vi "Sort_TC_Data.vi"(10 "TC_data":dbl[](array[numeric]), 11 "AlarmSettings":T1={"TC13"={"Enbl"=FALSE, "ErrsAndWarns"={0.0, 5.663716814159292, 7.168141592920354, 8.584070796460177}}, "AI1"={"Enbl"=FALSE, "ErrsAndWarns"={0.0, 5.663716814159292, 7.168141592920354, 8.584070796460177}}, "AI2"={"Enbl"=FALSE, "ErrsAndWarns"={0.0, 5.663716814159292, 7.168141592920354, 8.584070796460177}}, "AI3"={"Enbl"=FALSE, "ErrsAndWarns"={0.0, 5.663716814159292, 7.168141592920354, 8.584070796460177}}, "AI4"={"Enbl"=FALSE, "ErrsAndWarns"={0.0, 5.663716814159292, 7.168141592920354, 8.584070796460177}}, "AI5"={"Enbl"=FALSE, "ErrsAndWarns"={0.0, 5.663716814159292, 7.168141592920354, 8.584070796460177}}, "AI6"={"Enbl"=FALSE, "ErrsAndWarns"={0.0, 5.663716814159292, 7.168141592920354, 8.584070796460177}}, "AI18"={"Enbl"=FALSE, "ErrsAndWarns"={0.0, 5.663716814159292, 7.168141592920354, 8.584070796460177}}, "AI19"={"Enbl"=FALSE, "ErrsAndWarns"={0.0, 5.663716814159292, 7.168141592920354, 8.584070796460177}}, "TE1"={"Enbl"=FALSE, "ErrsAndWarns"={0.0, 5.663716814159292, 7.168141592920354, 8.584070796460177}}, "TE2"={"Enbl"=FALSE, "ErrsAndWarns"={0.0, 5.663716814159292, 7.168141592920354, 8.584070796460177}}, "TE3"={"Enbl"=FALSE, "ErrsAndWarns"={0.0, 5.663716814159292, 7.168141592920354, 8.584070796460177}}, "ADAM1"={"Enbl"=FALSE, "ErrsAndWarns"={0.0, 5.663716814159292, 7.168141592920354, 8.584070796460177}}, "ADAM2"={"Enbl"=FALSE, "ErrsAndWarns"={0.0, 5.663716814159292, 7.168141592920354, 8.584070796460177}}, "ADAM3"={"Enbl"=FALSE, "ErrsAndWarns"={0.0, 5.663716814159292, 7.168141592920354, 8.584070796460177}}, "ADAM4"={"Enbl"=FALSE, "ErrsAndWarns"={0.0, 5.663716814159292, 7.168141592920354, 8.584070796460177}}, "72CoBeacFreq"={"Enbl"=FALSE, "ErrsAndWarns"={0.0, 5.663716814159292, 7.168141592920354, 8.584070796460177}}, "72CoCalFreq"={"Enbl"=FALSE, "ErrsAndWarns"={0.0, 5.663716814159292, 7.168141592920354, 8.584070796460177}}, "84CoBeacFreq"={"Enbl"=FALSE, "ErrsAndWarns"={0.0, 5.663716814159292, 7.168141592920354, 8.584070796460177}}, "84CoCalFreq"={"Enbl"=FALSE, "ErrsAndWarns"={0.0, 5.663716814159292, 7.168141592920354, 8.584070796460177}}, "72Co_CalTonePwr"={"Enbl"=FALSE, "ErrsAndWarns"={0.0, 5.663716814159292, 7.168141592920354, 8.584070796460177}}, "72X_CalTonePwr"={"Enbl"=FALSE, "ErrsAndWarns"={0.0, 5.663716814159292, 7.168141592920354, 8.584070796460177}}, "84Co_CalTonePwr"={"Enbl"=FALSE, "ErrsAndWarns"={0.0, 5.663716814159292, 7.168141592920354, 8.584070796460177}}, "84X_CalTonePwr"={"Enbl"=FALSE, "ErrsAndWarns"={0.0, 5.663716814159292, 7.168141592920354, 8.584070796460177}}} {"84X_CalTonePwr"."ErrsAndWarns" scale=-120.0..-45.0; "72X_CalTonePwr"."ErrsAndWarns" scale=-120.0..-45.0; "84Co_CalTonePwr"."ErrsAndWarns" scale=-120.0..-45.0; "72Co_CalTonePwr"."ErrsAndWarns" scale=-120.0..-45.0; "84CoCalFreq"."ErrsAndWarns" scale=24.9..25.1; "84CoBeacFreq"."ErrsAndWarns" scale=25.5..27.0; "72CoCalFreq"."ErrsAndWarns" scale=24.9..25.1; "72CoBeacFreq"."ErrsAndWarns" scale=25.5..27.0; "ADAM4"."ErrsAndWarns" scale=30.0..52.0; "ADAM3"."ErrsAndWarns" scale=30.0..52.0; "ADAM2"."ErrsAndWarns" scale=30.0..52.0; "ADAM1"."ErrsAndWarns" scale=30.0..52.0; "TE3"."ErrsAndWarns" scale=30.0..52.0; "TE2"."ErrsAndWarns" scale=30.0..52.0; "TE1"."ErrsAndWarns" scale=20.0..52.0; "AI19"."ErrsAndWarns" scale=0.0..60.0; "AI18"."ErrsAndWarns" scale=-10.0..10.0; "AI6"."ErrsAndWarns" scale=0.0..35.0; "AI5"."ErrsAndWarns" scale=0.0..20.0; "AI4"."ErrsAndWarns" scale=0.0..15.0; "AI3"."ErrsAndWarns" scale=0.0..10.0; "AI2"."ErrsAndWarns" scale=0.0..10.0; "TC13"."ErrsAndWarns" scale=-10.0..40.0}) -> (3 "TC_Variant":variant)   [LabVIEW 2018]
uses:
  Controls/Clusts/AlarmSettingsClust.ctl
  Controls/Clusts/AlarmThresh_OneChan.ctl
  HDF5/TC_Data_Structure.ctl
  Controls/Clusts/All_TC_Error_Status.ctl
  Controls/Clusts/ErrorStatus.ctl
  Controls/Clusts/All_TC_Error_and_Data.ctl
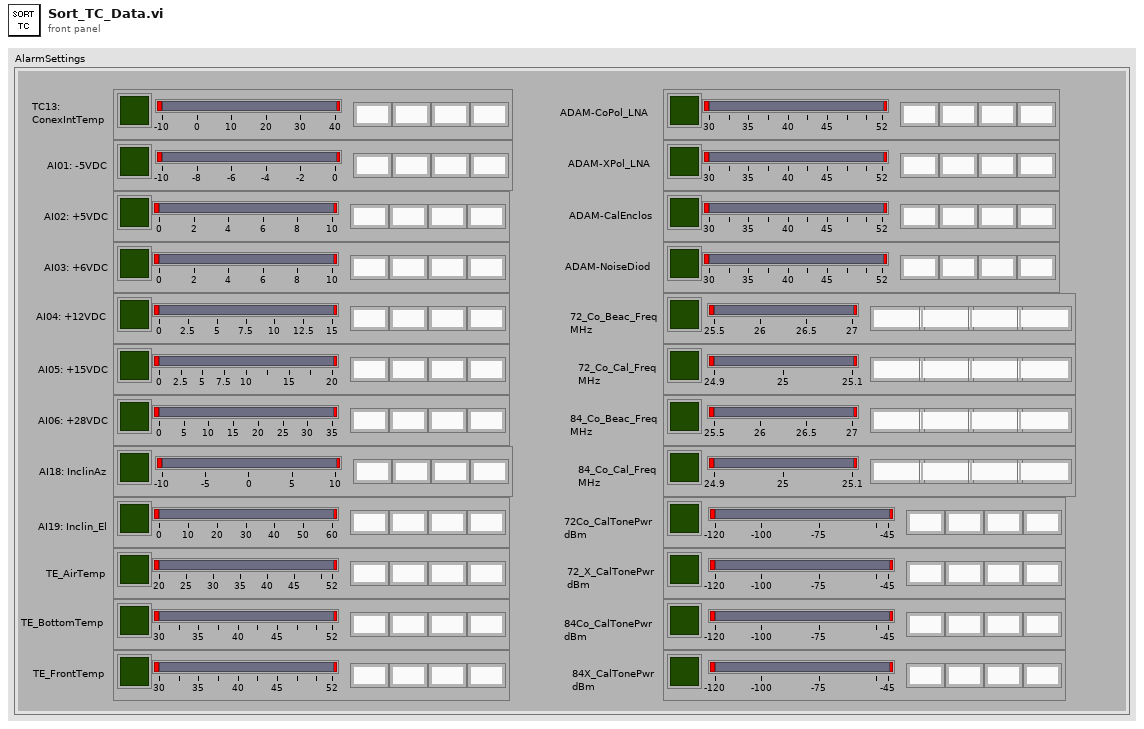
[diagram p1: front panel]
types:
  T1 = typedef "AlarmSettingsClust.ctl" = cluster{"TC13":T2, "AI1":T2, "AI2":T2, "AI3":T2, "AI4":T2, "AI5":T2, "AI6":T2, "AI18":T2, "AI19":T2, "TE1":T2, "TE2":T2, "TE3":T2, "ADAM1":T2, "ADAM2":T2, "ADAM3":T2, "ADAM4":T2, "72CoBeacFreq":T2, "72CoCalFreq":T2, "84CoBeacFreq":T2, "84CoCalFreq":T2, "72Co_CalTonePwr":T2, "72X_CalTonePwr":T2, "84Co_CalTonePwr":T2, "84X_CalTonePwr":T2}
  T2 = typedef "AlarmThresh_OneChan.ctl" = cluster{"Enbl":bool, "ErrsAndWarns":cluster{dbl, dbl, dbl, dbl}}
  T3 = typedef "All_TC_Error_and_Data.ctl" = cluster{"TCData":T4, "All_TC_ErrorStatus":T5}
  T4 = typedef "TC_Data_Structure.ctl" = cluster{"TimeStamp":dbl, "TimeString":string, "TC0_LP1_Hi":dbl, "TC1_LP1_MidHi":dbl, "TC2_LP1_Mid":dbl, "TC3_LP1_LoMid":dbl, "TC4_LP1_Lo":dbl, "TC5_LP2_Hi":dbl, "TC6_LP2_MidHi":dbl, "TC7_LP2_Mid":dbl, "TC8_LP2_LoMid":dbl, "TC9_LP2_Lo":dbl, "TC10_HVAC_Cond_In":dbl, "TC11_HVAC_Cond_Out":dbl, "TC12_Gen_Exhaust":dbl, "TC13_Amb_Inter":dbl, "TC14_Unused":dbl, "TC15_Unused":dbl, "TC16_Unused":dbl, "TC17_Unused":dbl, "TC18_Unused":dbl, "TC19_Unused":dbl, "TC20_Unused":dbl, "TC21_Unused":dbl, "TC22_Unused":dbl, "TC23_Unused":dbl, "TC24_Unused":dbl, "TC25_Unused":dbl, "TC26_Unused":dbl, "TC27_Unused":dbl, "TC28_Unused":dbl, "TC29_Unused":dbl, "TC30_Unused":dbl, "TC31_Unused":dbl}
  T5 = typedef "All_TC_Error_Status.ctl" = cluster{"TC 0":T6, "TC 1":T6, "TC 2":T6, "TC 3":T6, "TC 4":T6, "TC 5":T6, "TC 6":T6, "TC 7":T6, "TC 8":T6, "TC 9":T6, "TC 10":T6, "TC 11":T6, "TC 12":T6, "TC 13":T6, "TC 14":T6, "TC 15":T6, "TC 16":T6, "TC 17":T6, "TC 18":T6, "TC 19":T6, "TC 20":T6}
  T6 = typedef "ErrorStatus.ctl" = cluster{"RX?":bool, "Warn":bool, "Error":bool, "Enabl":bool, "Source":string}
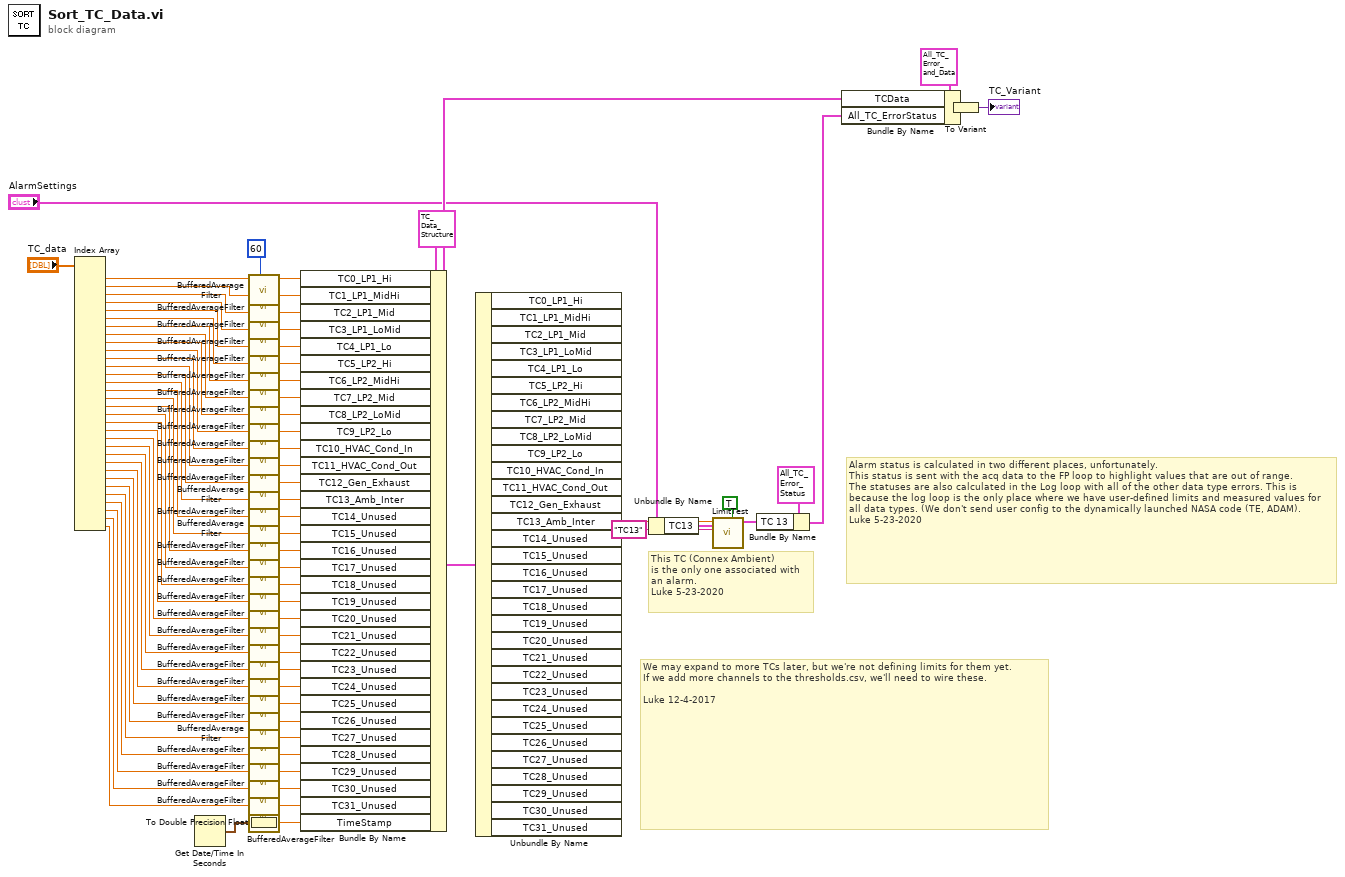
[diagram p0: block diagram]
diagram:
  w51 = 60 ("Buffer Size")
  # "This TC (Connex Ambient)\nis the only one associated with\nan alarm.\nLuke 5-23-2020"
  # "Alarm status is calculated in two different places, unfortunately.\nThis status is sent with the acq data to the FP loop to highlight values that are out of range.\nThe statuses are also calculated in the Log loop with all of the other data type errors. This is because the log loop is the only place where we have user-defined limits and measured values for all data types. (We don't send user config to the dynamically launched NASA code (TE, ADAM). \nLuke 5-23-2020"
  # "We may expand to more TCs later, but we're not defining limits for them yet.\nIf we add more channels to the thresholds.csv, we'll need to wire these.\n\nLuke 12-4-2017"
  n1 = Index Array(array="TC_data") -> (element #1=w70:dbl, element #2=w69:dbl, element #3=w68:dbl, element #4=w67:dbl, element #5=w66:dbl, element #6=w65:dbl, element #7=w64:dbl, element #8=w63:dbl, element #9=w62:dbl, element #10=w61:dbl, element #11=w60:dbl, element #12=w59:dbl, element #13=w58:dbl, element #14=w57:dbl, element #15=w56:dbl, element #16=w55:dbl, element #17=w54:dbl, element #18=w53:dbl, element #19=w52:dbl, element #20=w50:dbl, element #21=w49:dbl, element #22=w48:dbl, element #23=w47:dbl, element #24=w46:dbl, element #25=w45:dbl, element #26=w44:dbl, element #27=w43:dbl, element #28=w42:dbl, element #29=w41:dbl, element #30=w40:dbl, element #31=w39:dbl, element #32=w38:dbl)  [unwired: 32 in]
  n2 = Get Date/Time In Seconds() -> (seconds since 1Jan1904=w1:timestamp)
  n3 = call "BufferedAverageFilter.vi"("Buffer Size"=w51, "Signal"=w70) -> ("FilteredSignal"=w37:dbl)  [unwired: 9 in]
  n4 = call "BufferedAverageFilter.vi"("Buffer Size"=w51, "Signal"=w69) -> ("FilteredSignal"=w36:dbl)  [unwired: 9 in]
  n5 = call "BufferedAverageFilter.vi"("Buffer Size"=w51, "Signal"=w68) -> ("FilteredSignal"=w35:dbl)  [unwired: 9 in]
  n6 = call "BufferedAverageFilter.vi"("Buffer Size"=w51, "Signal"=w67) -> ("FilteredSignal"=w34:dbl)  [unwired: 9 in]
  n7 = call "BufferedAverageFilter.vi"("Buffer Size"=w51, "Signal"=w66) -> ("FilteredSignal"=w33:dbl)  [unwired: 9 in]
  n8 = call "BufferedAverageFilter.vi"("Buffer Size"=w51, "Signal"=w65) -> ("FilteredSignal"=w32:dbl)  [unwired: 9 in]
  n9 = call "BufferedAverageFilter.vi"("Buffer Size"=w51, "Signal"=w64) -> ("FilteredSignal"=w31:dbl)  [unwired: 9 in]
  n10 = call "BufferedAverageFilter.vi"("Buffer Size"=w51, "Signal"=w63) -> ("FilteredSignal"=w30:dbl)  [unwired: 9 in]
  n11 = call "BufferedAverageFilter.vi"("Buffer Size"=w51, "Signal"=w62) -> ("FilteredSignal"=w29:dbl)  [unwired: 9 in]
  n12 = call "BufferedAverageFilter.vi"("Buffer Size"=w51, "Signal"=w61) -> ("FilteredSignal"=w28:dbl)  [unwired: 9 in]
  n13 = call "BufferedAverageFilter.vi"("Buffer Size"=w51, "Signal"=w60) -> ("FilteredSignal"=w27:dbl)  [unwired: 9 in]
  n14 = call "BufferedAverageFilter.vi"("Buffer Size"=w51, "Signal"=w59) -> ("FilteredSignal"=w26:dbl)  [unwired: 9 in]
  n15 = call "BufferedAverageFilter.vi"("Buffer Size"=w51, "Signal"=w58) -> ("FilteredSignal"=w25:dbl)  [unwired: 9 in]
  n16 = call "BufferedAverageFilter.vi"("Buffer Size"=w51, "Signal"=w57) -> ("FilteredSignal"=w24:dbl)  [unwired: 9 in]
  n17 = call "BufferedAverageFilter.vi"("Buffer Size"=w51, "Signal"=w56) -> ("FilteredSignal"=w23:dbl)  [unwired: 9 in]
  n18 = call "BufferedAverageFilter.vi"("Buffer Size"=w51, "Signal"=w55) -> ("FilteredSignal"=w22:dbl)  [unwired: 9 in]
  n19 = call "BufferedAverageFilter.vi"("Buffer Size"=w51, "Signal"=w54) -> ("FilteredSignal"=w21:dbl)  [unwired: 9 in]
  n20 = call "BufferedAverageFilter.vi"("Buffer Size"=w51, "Signal"=w53) -> ("FilteredSignal"=w20:dbl)  [unwired: 9 in]
  n21 = call "BufferedAverageFilter.vi"("Buffer Size"=w51, "Signal"=w52) -> ("FilteredSignal"=w19:dbl)  [unwired: 9 in]
  n22 = call "BufferedAverageFilter.vi"("Buffer Size"=w51, "Signal"=w50) -> ("FilteredSignal"=w18:dbl)  [unwired: 9 in]
  n23 = call "BufferedAverageFilter.vi"("Buffer Size"=w51, "Signal"=w49) -> ("FilteredSignal"=w17:dbl)  [unwired: 9 in]
  n24 = call "BufferedAverageFilter.vi"("Buffer Size"=w51, "Signal"=w48) -> ("FilteredSignal"=w16:dbl)  [unwired: 9 in]
  n25 = call "BufferedAverageFilter.vi"("Buffer Size"=w51, "Signal"=w47) -> ("FilteredSignal"=w15:dbl)  [unwired: 9 in]
  n26 = call "BufferedAverageFilter.vi"("Buffer Size"=w51, "Signal"=w46) -> ("FilteredSignal"=w14:dbl)  [unwired: 9 in]
  n27 = call "BufferedAverageFilter.vi"("Buffer Size"=w51, "Signal"=w45) -> ("FilteredSignal"=w13:dbl)  [unwired: 9 in]
  n28 = call "BufferedAverageFilter.vi"("Buffer Size"=w51, "Signal"=w44) -> ("FilteredSignal"=w12:dbl)  [unwired: 9 in]
  n29 = call "BufferedAverageFilter.vi"("Buffer Size"=w51, "Signal"=w43) -> ("FilteredSignal"=w11:dbl)  [unwired: 9 in]
  n30 = call "BufferedAverageFilter.vi"("Buffer Size"=w51, "Signal"=w42) -> ("FilteredSignal"=w10:dbl)  [unwired: 9 in]
  n31 = call "BufferedAverageFilter.vi"("Buffer Size"=w51, "Signal"=w41) -> ("FilteredSignal"=w9:dbl)  [unwired: 9 in]
  n32 = call "BufferedAverageFilter.vi"("Buffer Size"=w51, "Signal"=w40) -> ("FilteredSignal"=w8:dbl)  [unwired: 9 in]
  n33 = call "BufferedAverageFilter.vi"("Buffer Size"=w51, "Signal"=w39) -> ("FilteredSignal"=w7:dbl)  [unwired: 9 in]
  n34 = call "BufferedAverageFilter.vi"("Buffer Size"=w51, "Signal"=w38) -> ("FilteredSignal"=w6:dbl)  [unwired: 9 in]
  n35 = To Double Precision Float(number=w1) -> (double precision float=w2:dbl)
  n36 = Bundle By Name(cluster=T4 {"TimeStamp"=0.0, "TimeString"="", "TC0_LP1_Hi"=0.0, "TC1_LP1_MidHi"=0.0, "TC2_LP1_Mid"=0.0, "TC3_LP1_LoMid"=0.0, "TC4_LP1_Lo"=0.0, "TC5_LP2_Hi"=0.0, "TC6_LP2_MidHi"=0.0, "TC7_LP2_Mid"=0.0, "TC8_LP2_LoMid"=0.0, "TC9_LP2_Lo"=0.0, "TC10_HVAC_Cond_In"=0.0, "TC11_HVAC_Cond_Out"=0.0, "TC12_Gen_Exhaust"=0.0, "TC13_Amb_Inter"=0.0, "TC14_Unused"=0.0, "TC15_Unused"=0.0, "TC16_Unused"=0.0, "TC17_Unused"=0.0, "TC18_Unused"=0.0, "TC19_Unused"=0.0, "TC20_Unused"=0.0, "TC21_Unused"=0.0, "TC22_Unused"=0.0, "TC23_Unused"=0.0, "TC24_Unused"=0.0, "TC25_Unused"=0.0, "TC26_Unused"=0.0, "TC27_Unused"=0.0, "TC28_Unused"=0.0, "TC29_Unused"=0.0, "TC30_Unused"=0.0, "TC31_Unused"=0.0} ("TCData"), "TC0_LP1_Hi"=w37, "TC1_LP1_MidHi"=w36, "TC2_LP1_Mid"=w35, "TC3_LP1_LoMid"=w34, "TC4_LP1_Lo"=w33, "TC5_LP2_Hi"=w32, "TC6_LP2_MidHi"=w31, "TC7_LP2_Mid"=w30, "TC8_LP2_LoMid"=w29, "TC9_LP2_Lo"=w28, "TC10_HVAC_Cond_In"=w27, "TC11_HVAC_Cond_Out"=w26, "TC12_Gen_Exhaust"=w25, "TC13_Amb_Inter"=w24, "TC14_Unused"=w23, "TC15_Unused"=w22, "TC16_Unused"=w21, "TC17_Unused"=w20, "TC18_Unused"=w19, "TC19_Unused"=w18, "TC20_Unused"=w17, "TC21_Unused"=w16, "TC22_Unused"=w15, "TC23_Unused"=w14, "TC24_Unused"=w13, "TC25_Unused"=w12, "TC26_Unused"=w11, "TC27_Unused"=w10, "TC28_Unused"=w9, "TC29_Unused"=w8, "TC30_Unused"=w7, "TC31_Unused"=w6, "TimeStamp"=w2) -> (w73:T4)
  n37 = Unbundle By Name(w73) -> ("TC13_Amb_Inter"=w77:dbl)  [unwired: 31 out]
  n38 = Unbundle By Name("AlarmSettings") -> ("TC13"=w78:T2)
  n39 = call "LimitTest.vi"("RX?"=TRUE, "AlarmCfg"=w78, "Source"="TC13", "Data"=w77) -> ("ErrorStatus"=w75:T6)  [unwired: 7 in]
  n40 = Bundle By Name(cluster=T5 {"TC 0"={"RX?"=FALSE, "Warn"=FALSE, "Error"=FALSE, "Enabl"=FALSE, "Source"=""}, "TC 1"={"RX?"=FALSE, "Warn"=FALSE, "Error"=FALSE, "Enabl"=FALSE, "Source"=""}, "TC 2"={"RX?"=FALSE, "Warn"=FALSE, "Error"=FALSE, "Enabl"=FALSE, "Source"=""}, "TC 3"={"RX?"=FALSE, "Warn"=FALSE, "Error"=FALSE, "Enabl"=FALSE, "Source"=""}, "TC 4"={"RX?"=FALSE, "Warn"=FALSE, "Error"=FALSE, "Enabl"=FALSE, "Source"=""}, "TC 5"={"RX?"=FALSE, "Warn"=FALSE, "Error"=FALSE, "Enabl"=FALSE, "Source"=""}, "TC 6"={"RX?"=FALSE, "Warn"=FALSE, "Error"=FALSE, "Enabl"=FALSE, "Source"=""}, "TC 7"={"RX?"=FALSE, "Warn"=FALSE, "Error"=FALSE, "Enabl"=FALSE, "Source"=""}, "TC 8"={"RX?"=FALSE, "Warn"=FALSE, "Error"=FALSE, "Enabl"=FALSE, "Source"=""}, "TC 9"={"RX?"=FALSE, "Warn"=FALSE, "Error"=FALSE, "Enabl"=FALSE, "Source"=""}, "TC 10"={"RX?"=FALSE, "Warn"=FALSE, "Error"=FALSE, "Enabl"=FALSE, "Source"=""}, "TC 11"={"RX?"=FALSE, "Warn"=FALSE, "Error"=FALSE, "Enabl"=FALSE, "Source"=""}, "TC 12"={"RX?"=FALSE, "Warn"=FALSE, "Error"=FALSE, "Enabl"=FALSE, "Source"=""}, "TC 13"={"RX?"=FALSE, "Warn"=FALSE, "Error"=FALSE, "Enabl"=FALSE, "Source"=""}, "TC 14"={"RX?"=FALSE, "Warn"=FALSE, "Error"=FALSE, "Enabl"=FALSE, "Source"=""}, "TC 15"={"RX?"=FALSE, "Warn"=FALSE, "Error"=FALSE, "Enabl"=FALSE, "Source"=""}, "TC 16"={"RX?"=FALSE, "Warn"=FALSE, "Error"=FALSE, "Enabl"=FALSE, "Source"=""}, "TC 17"={"RX?"=FALSE, "Warn"=FALSE, "Error"=FALSE, "Enabl"=FALSE, "Source"=""}, "TC 18"={"RX?"=FALSE, "Warn"=FALSE, "Error"=FALSE, "Enabl"=FALSE, "Source"=""}, "TC 19"={"RX?"=FALSE, "Warn"=FALSE, "Error"=FALSE, "Enabl"=FALSE, "Source"=""}, "TC 20"={"RX?"=FALSE, "Warn"=FALSE, "Error"=FALSE, "Enabl"=FALSE, "Source"=""}} ("AllErrorStatus"), "TC 13"=w75) -> (w72:T5)
  n41 = Bundle By Name(cluster=T3 {"TCData"={"TimeStamp"=0.0, "TimeString"="", "TC0_LP1_Hi"=0.0, "TC1_LP1_MidHi"=0.0, "TC2_LP1_Mid"=0.0, "TC3_LP1_LoMid"=0.0, "TC4_LP1_Lo"=0.0, "TC5_LP2_Hi"=0.0, "TC6_LP2_MidHi"=0.0, "TC7_LP2_Mid"=0.0, "TC8_LP2_LoMid"=0.0, "TC9_LP2_Lo"=0.0, "TC10_HVAC_Cond_In"=0.0, "TC11_HVAC_Cond_Out"=0.0, "TC12_Gen_Exhaust"=0.0, "TC13_Amb_Inter"=0.0, "TC14_Unused"=0.0, "TC15_Unused"=0.0, "TC16_Unused"=0.0, "TC17_Unused"=0.0, "TC18_Unused"=0.0, "TC19_Unused"=0.0, "TC20_Unused"=0.0, "TC21_Unused"=0.0, "TC22_Unused"=0.0, "TC23_Unused"=0.0, "TC24_Unused"=0.0, "TC25_Unused"=0.0, "TC26_Unused"=0.0, "TC27_Unused"=0.0, "TC28_Unused"=0.0, "TC29_Unused"=0.0, "TC30_Unused"=0.0, "TC31_Unused"=0.0}, "All_TC_ErrorStatus"={"TC 0"={"RX?"=FALSE, "Warn"=FALSE, "Error"=FALSE, "Enabl"=FALSE, "Source"=""}, "TC 1"={"RX?"=FALSE, "Warn"=FALSE, "Error"=FALSE, "Enabl"=FALSE, "Source"=""}, "TC 2"={"RX?"=FALSE, "Warn"=FALSE, "Error"=FALSE, "Enabl"=FALSE, "Source"=""}, "TC 3"={"RX?"=FALSE, "Warn"=FALSE, "Error"=FALSE, "Enabl"=FALSE, "Source"=""}, "TC 4"={"RX?"=FALSE, "Warn"=FALSE, "Error"=FALSE, "Enabl"=FALSE, "Source"=""}, "TC 5"={"RX?"=FALSE, "Warn"=FALSE, "Error"=FALSE, "Enabl"=FALSE, "Source"=""}, "TC 6"={"RX?"=FALSE, "Warn"=FALSE, "Error"=FALSE, "Enabl"=FALSE, "Source"=""}, "TC 7"={"RX?"=FALSE, "Warn"=FALSE, "Error"=FALSE, "Enabl"=FALSE, "Source"=""}, "TC 8"={"RX?"=FALSE, "Warn"=FALSE, "Error"=FALSE, "Enabl"=FALSE, "Source"=""}, "TC 9"={"RX?"=FALSE, "Warn"=FALSE, "Error"=FALSE, "Enabl"=FALSE, "Source"=""}, "TC 10"={"RX?"=FALSE, "Warn"=FALSE, "Error"=FALSE, "Enabl"=FALSE, "Source"=""}, "TC 11"={"RX?"=FALSE, "Warn"=FALSE, "Error"=FALSE, "Enabl"=FALSE, "Source"=""}, "TC 12"={"RX?"=FALSE, "Warn"=FALSE, "Error"=FALSE, "Enabl"=FALSE, "Source"=""}, "TC 13"={"RX?"=FALSE, "Warn"=FALSE, "Error"=FALSE, "Enabl"=FALSE, "Source"=""}, "TC 14"={"RX?"=FALSE, "Warn"=FALSE, "Error"=FALSE, "Enabl"=FALSE, "Source"=""}, "TC 15"={"RX?"=FALSE, "Warn"=FALSE, "Error"=FALSE, "Enabl"=FALSE, "Source"=""}, "TC 16"={"RX?"=FALSE, "Warn"=FALSE, "Error"=FALSE, "Enabl"=FALSE, "Source"=""}, "TC 17"={"RX?"=FALSE, "Warn"=FALSE, "Error"=FALSE, "Enabl"=FALSE, "Source"=""}, "TC 18"={"RX?"=FALSE, "Warn"=FALSE, "Error"=FALSE, "Enabl"=FALSE, "Source"=""}, "TC 19"={"RX?"=FALSE, "Warn"=FALSE, "Error"=FALSE, "Enabl"=FALSE, "Source"=""}, "TC 20"={"RX?"=FALSE, "Warn"=FALSE, "Error"=FALSE, "Enabl"=FALSE, "Source"=""}}}, "TCData"=w73, "All_TC_ErrorStatus"=w72) -> (w71:T3)
  n42 = To Variant(anything=w71) -> (Variant=→"TC_Variant":variant)
